vi "SetControlPaneDeferUpdates.vi"(7 "Front Panel":refnum<vi>, 8 "error in (no error)":errorcluster, 9 "Defer Panel Updates":bool, 10 "Control Label":string, 11 "CtlLookup In":T1) -> (0 "error out":errorcluster, 2 "Front Panel Out":refnum<vi>, 3 "CtlLookup Out":T1)   [LabVIEW 2020, in "CtlReferences_API.lvlib"]
doc: "Defers updates for the panel of the specified control.\nIf the \"Front Panel\" reference is specified, the ctllookup is not performed."
uses:
  CtlReferences_API.lvlib
  CtlReferences/TypeDefs/CtlLookup.ctl
  CtlReferences/CtlReferences.lvclass
  CtlReferences/Get_OwningVIPanel.vi
  CtlReferences/GetCtlRef.vi
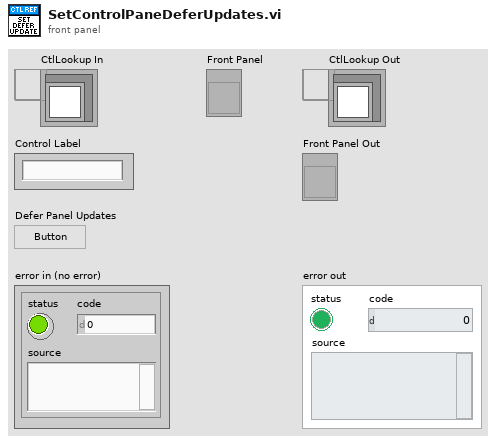
[diagram p1: front panel]
types:
  T1 = typedef "CtlReferences.lvlib/CtlReferences.lvclass/CtlLookup.ctl" = refnum<data-value>
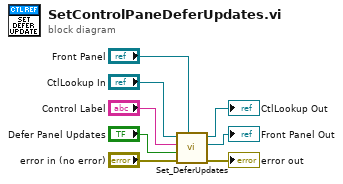
[diagram p0: block diagram]
diagram:
  n1 = call "Set_DeferUpdates.vi"("Front Panel"="Front Panel", "error in (no error)"="error in (no error)", "Defer Panel Updates"="Defer Panel Updates", "Control Label"="Control Label", "CtlLookup In"="CtlLookup In") -> ("error out"=→"error out":errorcluster, "Front Panel Out"=→"Front Panel Out":refnum<vi>, "CtlLookup Out"=→"CtlLookup Out":T1)  [unwired: 4 in]
